vi "start_binned.vi"   [LabVIEW 2015]
uses:
  phlib.dll
types:
  T1 = cluster{"initialized":bool, "devidx":i32, "Ch0 Level":i32, "Ch0 ZeroX":i32, "Ch1 Level":i32, "Ch1 ZeroX":i32, "sync rate":i32, "resolution":i32, "acq time":i32, "acq rate":i32, "# bins":u32, "Bin size":enum16{"1", "2", "4", "8", "16", "32", "64", "128"}, "min photons":u32, "truncate":u32}
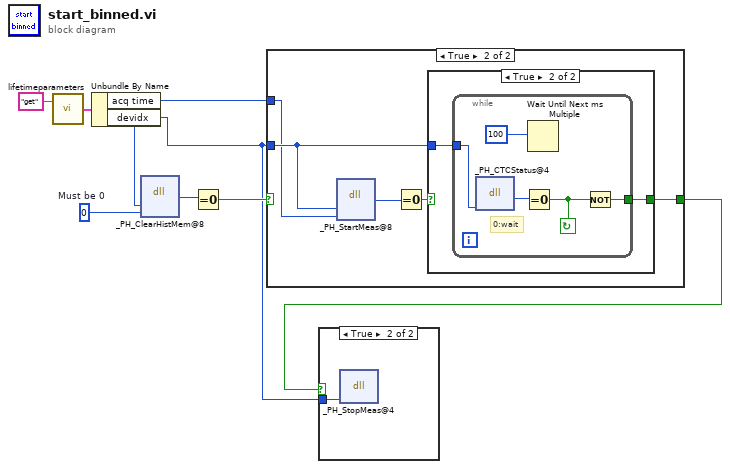
[diagram p0: block diagram]
diagram:
  w5 = 0  # Must be 0
  n1 = call "lifetimeparameters.vi"("command"="get") -> ("Params out"=w3:T1)  [unwired: 1 in]
  n2 = Unbundle By Name(w3) -> ("acq time"=w1:i32, "devidx"=w2:i32)
  n3 = dll-call lib="phlib.dll" fn="_PH_ClearHistMem@8" label="PH_ClearHistMem"("devidx"=w2, "block"=w5) -> (w7:i32)  [unwired: 5 in, 2 out]
  n4 = Equal To 0?(x=w7) -> (x = 0?=w6:bool)
  n5 = case shown="True" w6 {
    selector: w6 -> [w9 _]
    tunnel: [w9 w12] -> w8
    tunnel: w2 -> [_ w11]
    tunnel: w1 -> [_ w10]
    frame False {
    }
    frame True {
      n6 = dll-call lib="phlib.dll" fn="_PH_StartMeas@8" label="PH_StartMeas"("devidx"=w11, "tacq"=w10) -> (w14:i32)  [unwired: 5 in, 2 out]
      n7 = Equal To 0?(x=w14) -> (x = 0?=w13:bool)
      n8 = case shown="True" w13 {
        selector: w13 -> [w15 _]
        tunnel: [w15 w17] -> w12
        tunnel: w11 -> [_ w16]
        frame False {
        }
        frame True {
          n9 = while {
            tunnel: w16 -> [w18]
            tunnel: [w19] -> w17
            stop <- w20 continue-if-true
            # "0:wait"
            n10 = dll-call lib="phlib.dll" fn="_PH_CTCStatus@4" label="PH_CTCStatus"("devidx"=w18) -> (w22:i32)  [unwired: 4 in, 2 out]
            n11 = Equal To 0?(x=w22) -> (x = 0?=w20:bool)
            n12 = Wait Until Next ms Multiple(millisecond multiple=u32 100) -> ()  [unwired: 1 out]
            n13 = Not(x=w20) -> (.not. x?=w19:bool)
          }
        }
      }
    }
  }
  n14 = case shown="True" w8 {
    tunnel: w2 -> [_ w23]
    frame False {
    }
    frame True {
      n15 = dll-call lib="phlib.dll" fn="_PH_StopMeas@4" label="PH_StopMeas"("devidx"=w23) -> ()  [unwired: 5 in, 2 out]
    }
  }
